vi "GetConfig.vi"(8 "error in (no error)":errorcluster, 11 "Device in":refnum<class "Device.lvclass">) -> (0 "error out":errorcluster, 2 "Resp":string, 3 "Device out":refnum<class "Device.lvclass">)   [LabVIEW 2012, in "Device.lvclass"]
uses:
  Device.lvclass
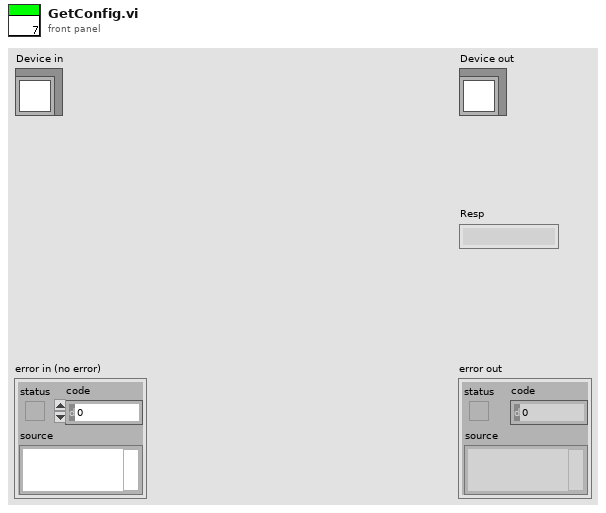
[diagram p1: front panel]
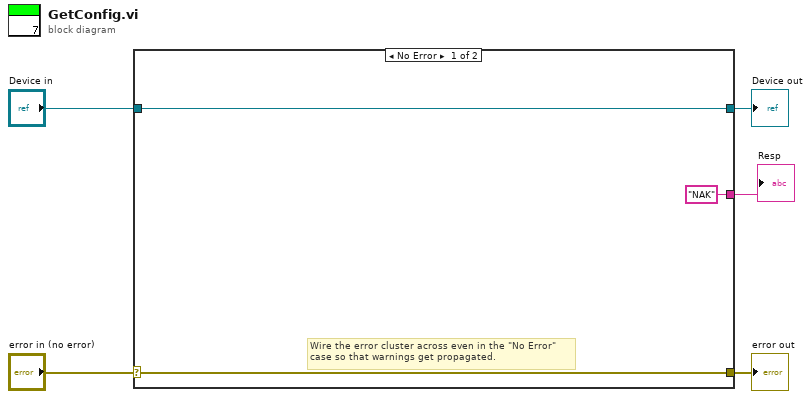
[diagram p0: block diagram]
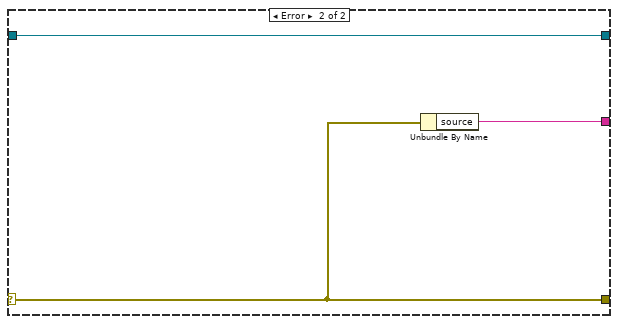
[diagram p2: hidden frame]
diagram:
  n1 = case shown="No Error" "error in (no error)" {
    selector: "error in (no error)" -> [w7 w10]
    tunnel: [w7 w10] -> w4
    tunnel: [w8 w11] -> w2
    tunnel: "Device in" -> [w8 w11]
    tunnel: ["NAK" ("source") w9] -> w1
    frame No Error {
      # "Wire the error cluster across even in the \"No Error\"\ncase so that warnings get propagated."
    }
    frame Error {
      n2 = Unbundle By Name(w10) -> ("source"=w9:string)
    }
  }
  "error out" <- w4
  "Device out" <- w2
  "Resp" <- w1
